vi "Check new DelayFormula and Update Delays.vi"(7 "Update HW":bool, 8 "error in (no error)":errorcluster, 9 "Delay Formula":string, 10 "ChnlName":string, 11 "BME_DG_System in":refnum<class "BME_DG_System.lvclass">) -> (0 "error out":errorcluster, 2 "Problem Chnls out":string[](array[string]), 3 "BME_DG_System out":refnum<class "BME_DG_System.lvclass">)   [LabVIEW 2009, in "POLARIS BME DG.lvlib" / "BME_DG_System.lvclass"]
uses:
  BME_DG_System.lvclass
  BME_DG_Chnl/BME_DG_Chnl.lvclass
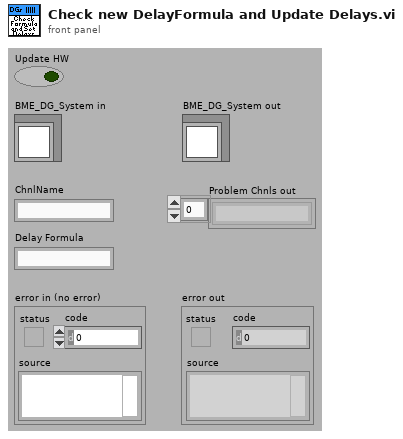
[diagram p1: front panel]
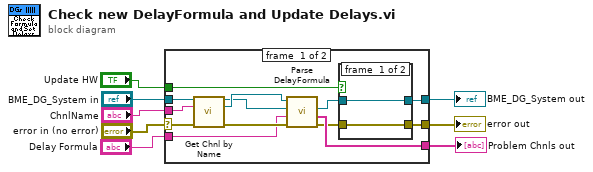
[diagram p0: block diagram]
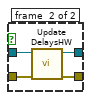
[diagram p2: hidden frame]
diagram:
  n1 = case shown="No Error" "error in (no error)" {
    selector: "error in (no error)" -> [w19 w29]
    tunnel: [w10 w29] -> w7
    tunnel: [w12 w28] -> w5
    tunnel: "BME_DG_System in" -> [w21 w28]
    tunnel: "ChnlName" -> [w20 _]
    tunnel: "Delay Formula" -> [w16 _]
    tunnel: [w14 _] -> w2
    tunnel: "Update HW" -> [w9 _]
    frame #0 {
      n2 = call "Get Chnl by Name.vi"("BME_DG_System in"=w21, "Chnl Name"=w20, "error in (no error)"=w19) -> ("BME_DG_System out"=w15:refnum<class "BME_DG_System.lvclass">, "BME_DG_Chnl"=w18:refnum<class "BME_DG_Chnl.lvclass">, "error out"=w17:errorcluster)  [unwired: 7 in, 3 out]
      n3 = call "Parse DelayFormula.vi"("error in (no error)"=w17, "DelayFormula"=w16, "BME_DG_System"=w15, "BME_DG_Chnl in"=w18) -> ("error out"=w11:errorcluster, "Problem Chnls out"=w14:string[], "BME_DG_System out"=w13:refnum<class "BME_DG_System.lvclass">)  [unwired: 5 in]
      n4 = case shown="True" w9 {
        tunnel: w13 -> [w23 w27]
        tunnel: [w23 w26] -> w12
        tunnel: w11 -> [w22 w25]
        tunnel: [w22 w24] -> w10
        frame #0 {
        }
        frame #1 {
          n5 = call "Update DelaysHW.vi"("error in (no error)"=w25, "BME_DG_System in"=w27) -> ("error out"=w24:errorcluster, "BME_DG_System out"=w26:refnum<class "BME_DG_System.lvclass">)  [unwired: 8 in]
        }
      }
    }
    frame #1 {
    }
  }
  "error out" <- w7
  "BME_DG_System out" <- w5
  "Problem Chnls out" <- w2
